vi "En_Disen_output.vi"(8 "error in (no error)":errorcluster, 10 "newstate":bool, 11 "VISA resource in":refnum<visa-resource-name>) -> (0 "error out":errorcluster, 2 "actual_state":bool, 3 "VISA resource out":refnum<visa-resource-name>)   [LabVIEW 2014, in "B&K Precision 9120 series.lvclass"]
uses:
  B&K Precision 9120 series.lvclass
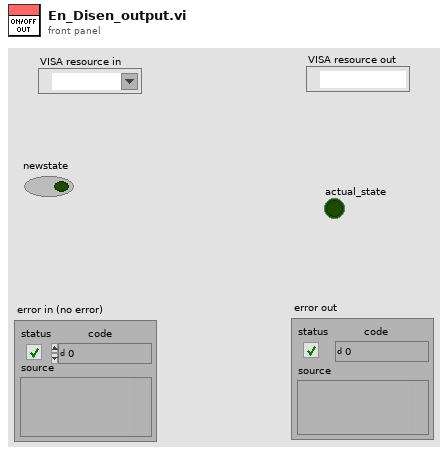
[diagram p1: front panel]
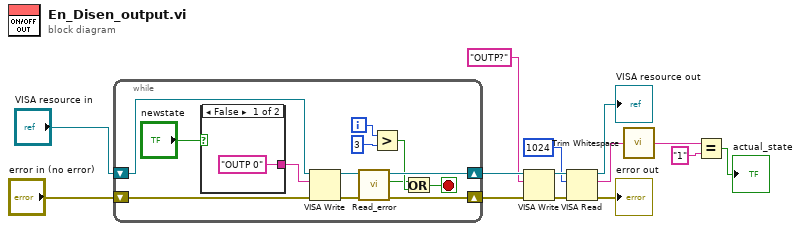
[diagram p0: block diagram]
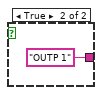
[diagram p2: hidden frame]
diagram:
  n1 = while {
    shift-right: [w23] -> w12
    shift-left: "VISA resource in" -> [w27]
    shift-right: [w22] -> w10
    shift-left: "error in (no error)" -> [w26]
    i -> [w18]
    stop <- w19 stop-if-true
    n2 = case shown="False" "newstate" {
      tunnel: ["OUTP 0" ("write buffer") "OUTP 1" ("write buffer")] -> w16
      frame False {
      }
      frame True {
      }
    }
    n3 = VISA Write(VISA resource name=w27, write buffer=w16, error in (no error)=w26) -> (VISA resource name out=w25:refnum<visa-resource-name>, error out=w24:errorcluster)  [unwired: 1 out]
    n4 = call "Read_error.vi"("error in (no error)"=w24, "VISA resource in"=w25) -> ("error out"=w22:errorcluster, "OK"=w17:bool, "VISA resource out"=w23:refnum<visa-resource-name>)  [unwired: 7 in]
    n5 = Greater?(x=w18, y=3) -> (0:w21:bool)
    n6 = Or(x=w17, y=w21) -> (x .or. y?=w19:bool)
  }
  n7 = VISA Write(VISA resource name=w12, write buffer="OUTP?", error in (no error)=w10) -> (VISA resource name out=w9:refnum<visa-resource-name>, error out=w8:errorcluster)  [unwired: 1 out]
  n8 = VISA Read(VISA resource name=w9, byte count=u32 1024, error in (no error)=w8) -> (VISA resource name out=→"VISA resource out":refnum<visa-resource-name>, read buffer=w4:string, error out=→"error out":errorcluster)  [unwired: 1 out]
  n9 = call <vilib>:"Trim Whitespace.vi"("string"=w4) -> ("trimmed string"=w2:string)  [unwired: 1 in]
  n10 = Equal?(x=w2, y="1") -> (x = y?=→"actual_state":bool)
